vi "点到行列(数组).vi"(8 "error in (no error)":errorcluster caption="错误输入（无错误）", 10 "坐标":T1, 11 "引用":refnum<vi>) -> (0 "error out":errorcluster caption="错误输出", 2 "数组坐标":cluster{"行":i32, "列":i32}, 3 "引用输出":refnum<vi>)   [LabVIEW 2014, in "表格.lvlib"]
uses:
  <vilib>/Utility/miscctls.llb/LVPoint32TypeDef.ctl
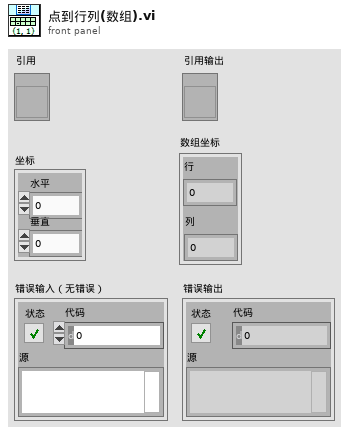
[diagram p1: front panel]
types:
  T1 = typedef "LVPoint32TypeDef.ctl" = cluster{"Horizontal":i32, "Vertical":i32}
  T2 = typedef "控件位置.ctl" = cluster{"左":i32, "上":i32, "右":i32, "下":i32}
  T3 = typedef "行列.ctl" = cluster{"行":i32, "列":i32}
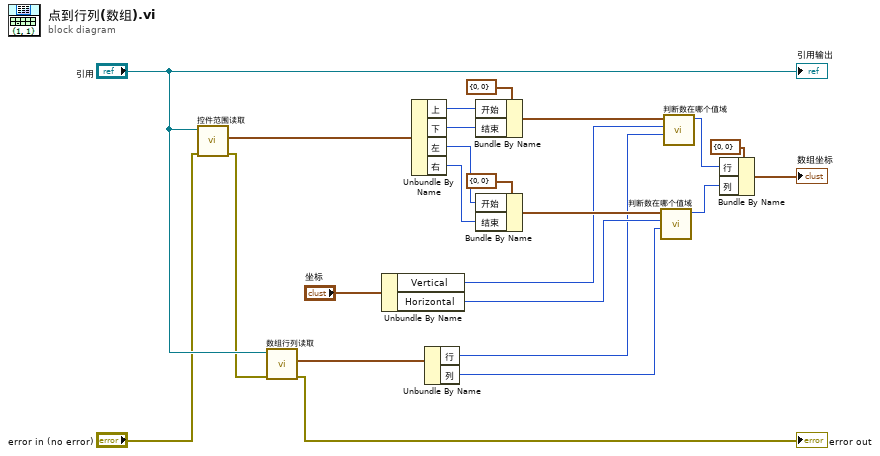
[diagram p0: block diagram]
diagram:
  n1 = call "控件范围读取.vi"("错误输入"="error in (no error)", "引用"="引用") -> ("错误输出"=w2:errorcluster, "坐标输出"=w5:T2)  [unwired: 7 in, 1 out]
  n2 = call "数组行列读取.vi"("错误输入（无错误）"=w2, "引用"="引用") -> ("错误输出"=→"error out":errorcluster, "行列"=w4:T3)  [unwired: 7 in, 1 out]
  n3 = Unbundle By Name("坐标") -> ("Vertical"=w10:i32, "Horizontal"=w9:i32)
  n4 = Unbundle By Name(w5) -> ("上"=w19:i32, "下"=w18:i32, "左"=w12:i32, "右"=w11:i32)
  n5 = Unbundle By Name(w4) -> ("行"=w8:i32, "列"=w7:i32)
  n6 = Bundle By Name(cluster=cluster{"开始":i32, "结束":i32} {"开始"=0, "结束"=0} ("首和尾"), "开始"=w19, "结束"=w18) -> (w17:cluster{"开始":i32, "结束":i32})
  n7 = Bundle By Name(cluster=cluster{"开始":i32, "结束":i32} {"开始"=0, "结束"=0} ("首和尾"), "开始"=w12, "结束"=w11) -> (w16:cluster{"开始":i32, "结束":i32})
  n8 = call-poly "判断数在哪个值域.vi"("平分数"=w7, "值"=w9, "首和尾"=w16) -> ("对应部分"=w14:i32)  [unwired: 8 in]
  n9 = call-poly "判断数在哪个值域.vi"("平分数"=w8, "值"=w10, "首和尾"=w17) -> ("对应部分"=w15:i32)  [unwired: 8 in]
  n10 = Bundle By Name(cluster=cluster{"行":i32, "列":i32} {"行"=0, "列"=0} ("数组坐标"), "行"=w15, "列"=w14) -> (→"数组坐标":cluster{"行":i32, "列":i32})
  "引用输出" <- "引用"
